vi "New Save.vi"() -> ()   [LabVIEW 2017]
panel:
  out "Waveform Graph 3":dynamicdata(graph)
  out "Waveform Graph 2":dynamicdata(graph)
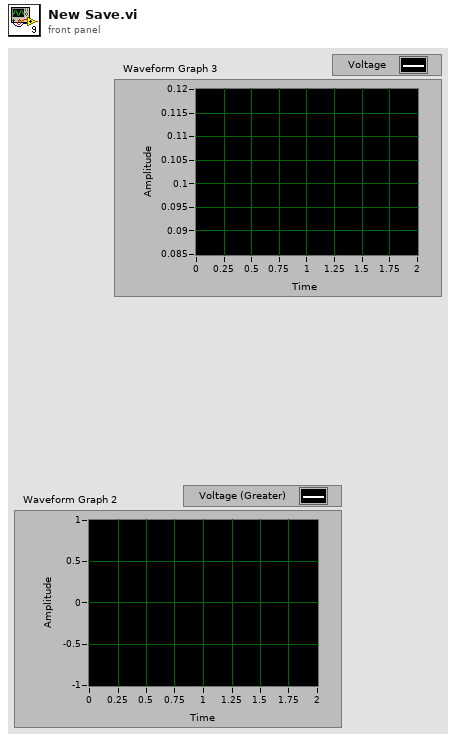
[diagram p1: front panel]
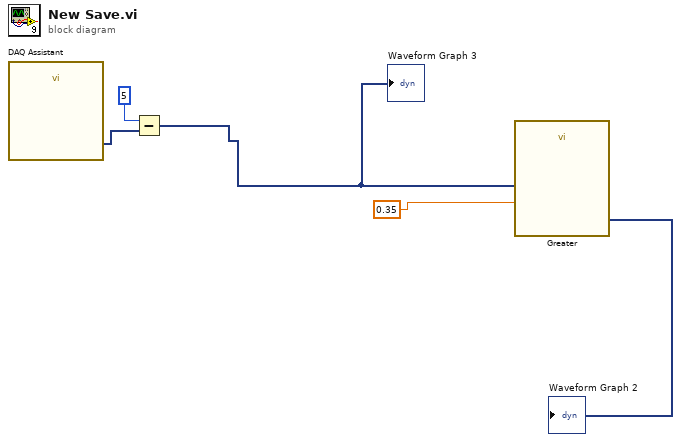
[diagram p0: block diagram]
diagram:
  n1 = call "DAQ Assistant"() -> ("data"=w2:dynamicdata)  [unwired: 17 in, 2 out]
  n2 = Subtract(x=5, y=w2) -> (x-y=w1:dynamicdata)
  "Waveform Graph 3" <- w1
  n3 = call "Greater"("Constant Value to Compare Against"=0.35, "Operand 1"=w1) -> ("Result"=→"Waveform Graph 2":dynamicdata)  [unwired: 8 in, 1 out]
